vi "GOOPUtil_GetClassName.vi"(0 "LabVIEW Object":refnum<class>, 5 "error in (no error)":errorcluster) -> (15 "IsEmptyObject?":bool, 16 "Class Name":string, 17 "lvlib Hierarchy":string[](array[string]), 18 "Full Class Name":string, 19 "error out":errorcluster)   [LabVIEW 2020, in "GOOPUtility.lvlib"]
doc: "Returns the name of the class, the lvlib hierarchy (if any) and the name space path of the class.\n\nThis is a collection of generic GOOP utility VIs. Please notice that it is important that the frontpanel of the Create, Destroy and GetObjectStatus is not removed when building an application."
uses:
  <vilib>/addons/GOOPUtility/GOOPUtility.lvlib
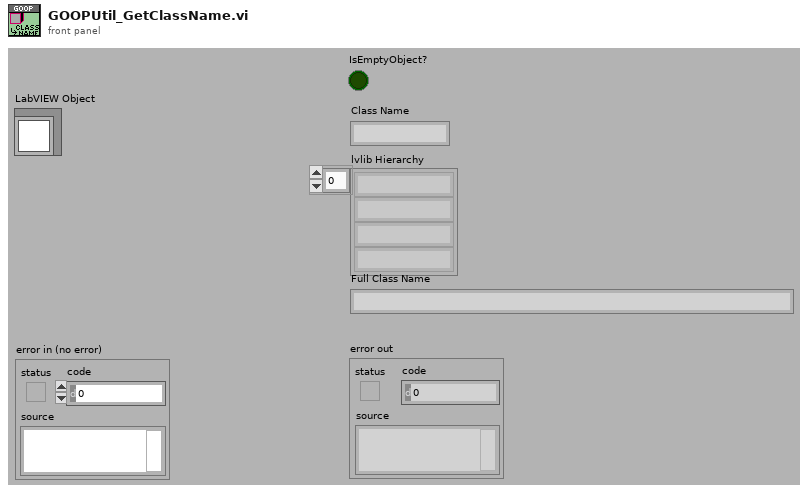
[diagram p1: front panel]
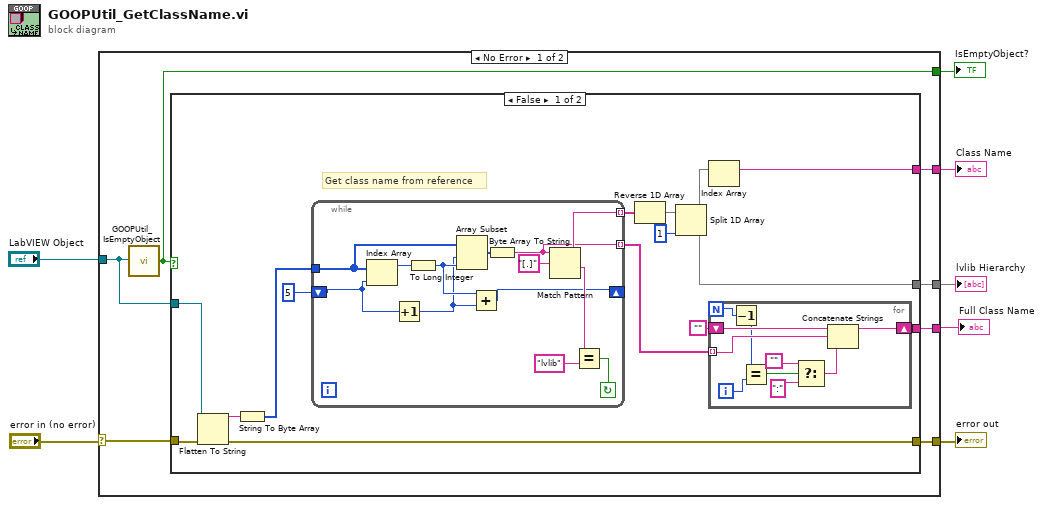
[diagram p0: block diagram]
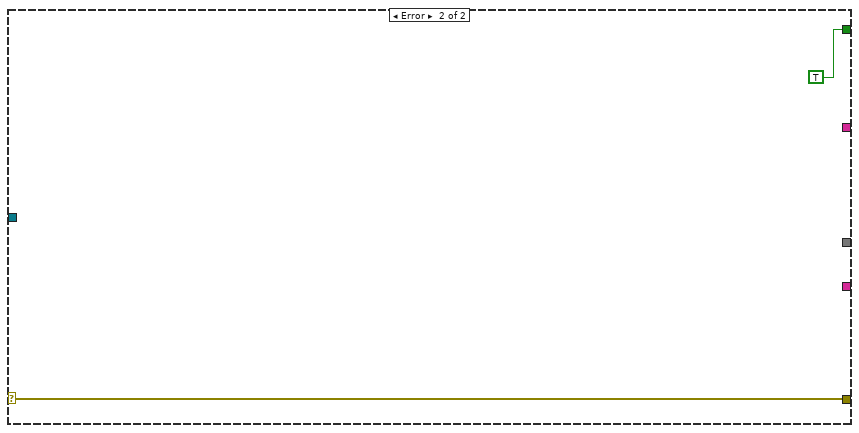
[diagram p3: hidden frame]
diagram:
  n1 = case shown="No Error" "error in (no error)" {
    selector: "error in (no error)" -> [w10 w55]
    tunnel: [w8 w55] -> w7
    tunnel: [w14 _] -> w6
    tunnel: "LabVIEW Object" -> [w9 _]
    tunnel: [w13 _] -> w3
    tunnel: [w12 _] -> w2
    tunnel: [w11 TRUE] -> w1
    frame No Error {
      n2 = call <vilib>:"GOOPUtil_IsEmptyObject.vi"("LabVIEW Object"=w9) -> ("IsEmpty?"=w11:bool)
      n3 = case shown="False" w11 {
        tunnel: [w28 _] -> w14
        tunnel: [w24 _] -> w13
        tunnel: [w21 _] -> w12
        tunnel: w10 -> [w18 w53]
        tunnel: w9 -> [w17 _]
        tunnel: [w15 w53] -> w8
        frame False {
          # "Get class name from reference"
          n4 = Flatten To String(anything=w17, error in (no error)=w18) -> (data string=w19:string, error out=w15:errorcluster)  [unwired: 2 in, 1 out]
          n5 = String To Byte Array(string=w19) -> (unsigned byte array=w16:u8[])
          n6 = while {
            tunnel: w16 -> [w52]
            shift-right: [w42] -> _
            shift-left: 5 ("index") -> [w45]
            tunnel: [w41] -> w23 mode=indexing
            tunnel: [w40] -> w20 mode=indexing
            stop <- w46 continue-if-true
            n7 = Index Array(array=w52, index=w45) -> (element=w51:u8)
            n8 = Increment(x=w45) -> (x+1=w43:i32)
            n9 = To Long Integer(number=w51) -> (32bit integer=w44:i32)
            n10 = Array Subset(array=w52, index=w43, length=w44) -> (w50:u8[])
            n11 = Add(x=w44, y=w43) -> (x+y=w42:i32)
            n12 = Byte Array To String(unsigned byte array=w50) -> (string=w40:string)
            n13 = Match Pattern(string=w40, regular expression="[.]") -> (before substring=w41:string, after substring=w48:string)  [unwired: 1 in, 2 out]
            n14 = Equal?(x=w48, y="lvlib") -> (x = y?=w46:bool)
          }
          n15 = Reverse 1D Array(array=w23) -> (reversed array=w27:string[])
          n16 = Split 1D Array(array=w27, index=1) -> (first subarray=w25:string[], second subarray=w24:string[])
          n17 = Index Array(array=w25) -> (element=w28:string)  [unwired: 1 in]
          n18 = for {
            N -> [w36]
            tunnel: w20 -> [w37] mode=indexing
            shift-right: [w38] -> w21
            shift-left: "" -> [w39]
            i -> [w35]
            n19 = Decrement(x=w36) -> (x-1=w34:i32)
            n20 = Equal?(x=w34, y=w35) -> (x = y?=w33:bool)
            n21 = Select(t="", s=w33, f=":" ("string")) -> (s? t:f=w31:string)
            n22 = Concatenate Strings(w39, w37, w31) -> (w38:string)
          }
        }
        frame True {
        }
      }
    }
    frame Error {
    }
  }
  "error out" <- w7
  "Class Name" <- w6
  "lvlib Hierarchy" <- w3
  "Full Class Name" <- w2
  "IsEmptyObject?" <- w1
